vi "FPGACentreReadout.vi"() -> ()   [LabVIEW 2018]
uses:
  State.ctl
  Data.ctl
  <vilib>/rvi/Emulation/niFpgaGetClockAttributes.vi
  <vilib>/rvi/Emulation/niFpgaSctlEmulationGetInTimedLoop.vi
  <vilib>/rvi/Emulation/niFpgaEmulationReportErrorSimple.vi
  <vilib>/rvi/Emulation/niFpgaProcessEmulError.vi
  <vilib>/rvi/eio/common/nirviEmuTemplateMethod_errors.vi
  <vilib>/rvi/Emulation/niFpgaCriticalErrorInLSC.vi
  <vilib>/eio/EIONode/EIONode.xnode
panel:
  out "Boolean":bool
  in  "PowerDown? 3":bool
  out "Data 3":i32
  in  "Gain/ChannelSelect 3":T1(ring)
  out "ConnectorA/DIO4":bool
  out "State 3":T2
  out "Data array3":i32[](array[numeric])
  in  "PowerDown? 2":bool
  out "Data 2":i32
  in  "Gain/ChannelSelect 2":T1(ring)
  out "ConnectorA/DIO2":bool
  out "State 2":T2
  out "Data array 2":i32[](array[numeric])
  out "RawCurrent":u16
  out "RawVoltage":i16
  out "State":T2
  out "ConnectorA/DIO0":bool
  out "Data array":i32[](array[numeric])
  in  "PowerDown?":bool
  out "Data":i32
  in  "Gain/ChannelSelect":T1(ring)
  in  "stop":bool
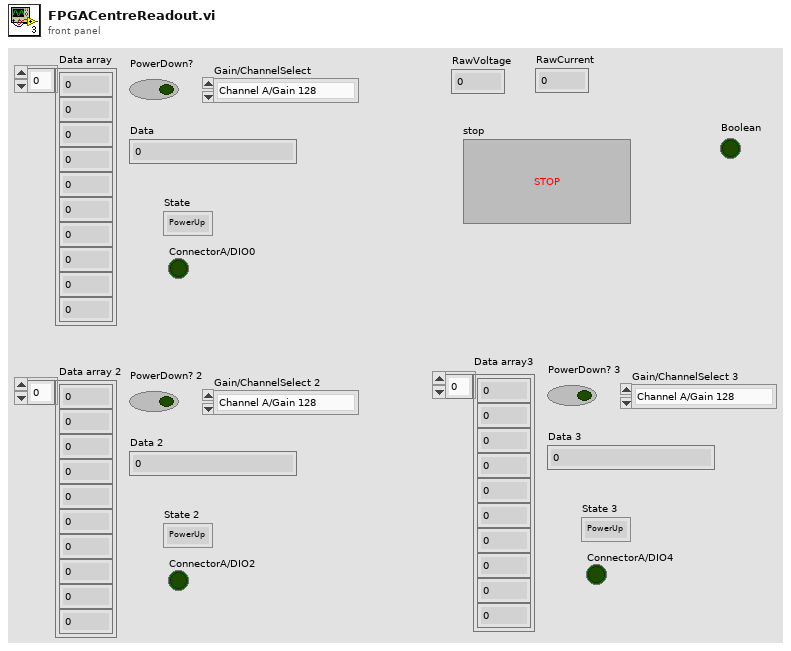
[diagram p1: front panel]
types:
  T1 = enum16{"Channel A/Gain 128", "Channel A/Gain 64", "Channel B/Gain 32"}
  T2 = typedef "State.ctl" = enum16{"PowerUp", "PowerDown", "Gain/ChannelSelect", "ReadData", "ClockLow", "ClockHigh", "ConvertData", "RetrievalReady?"}
  T3 = typedef "Data.ctl" = cluster{"DT":bool, "SCK":bool, "2's Data":i32, "PulseCount":u8, "DelayTime":u8, "Data":i32, "PowerDown?":bool, "Gain/ChannelSelect":enum16{"Channel A/Gain 128", "Channel A/Gain 64", "Channel B/Gain 32"}}
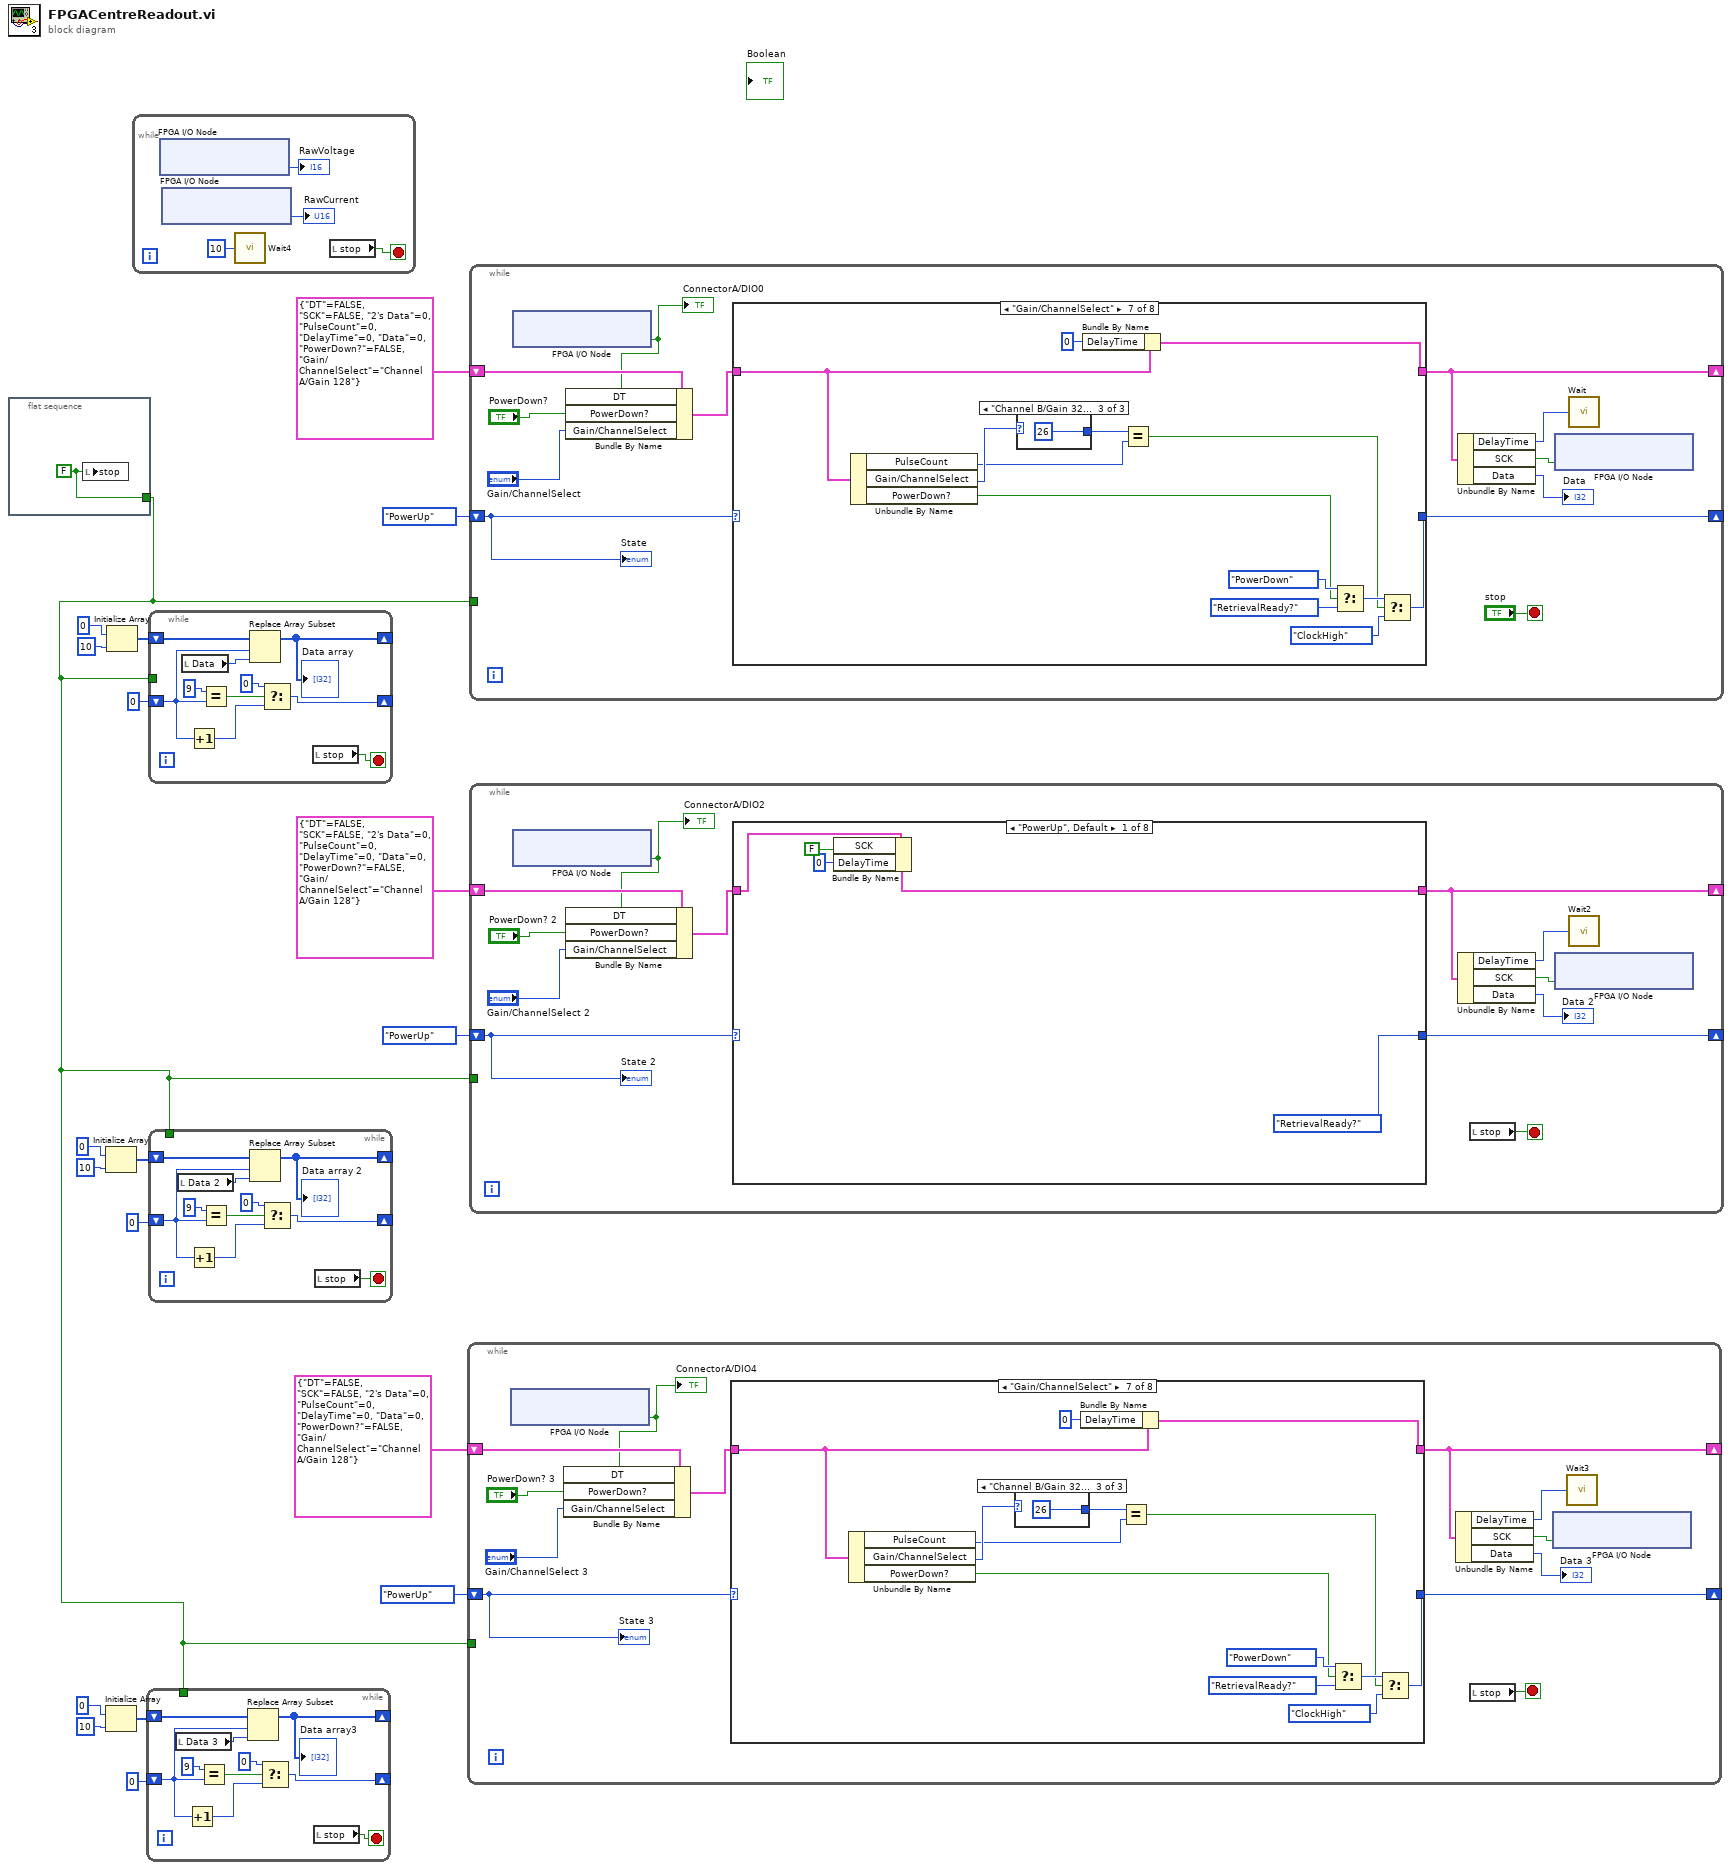
[diagram p0: block diagram]
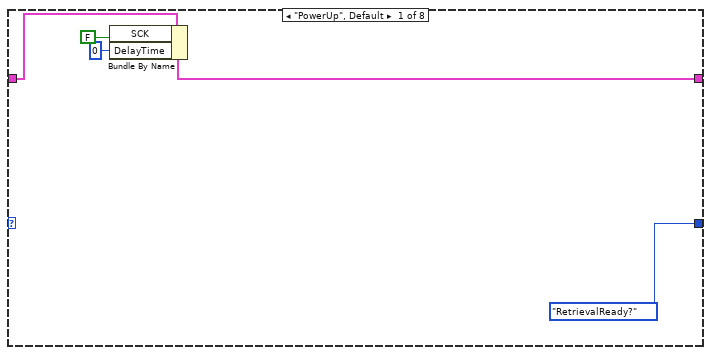
[diagram p2: hidden frame]
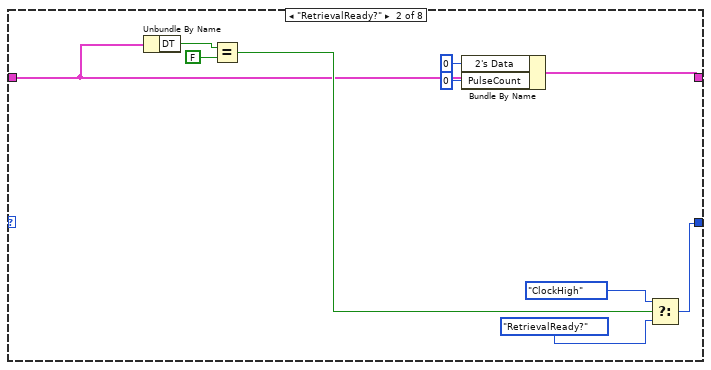
[diagram p3: hidden frame]
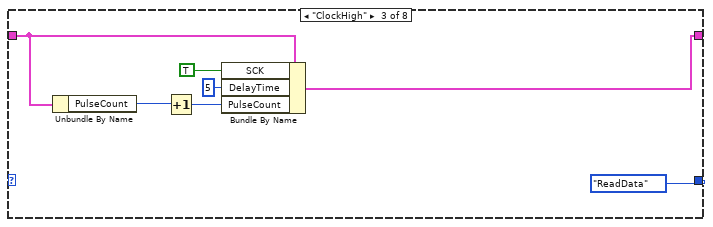
[diagram p4: hidden frame]
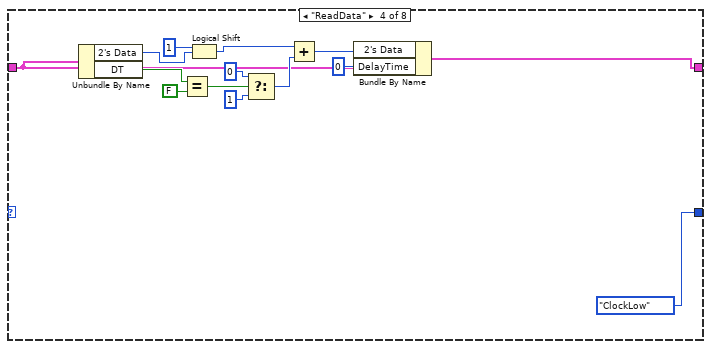
[diagram p5: hidden frame]
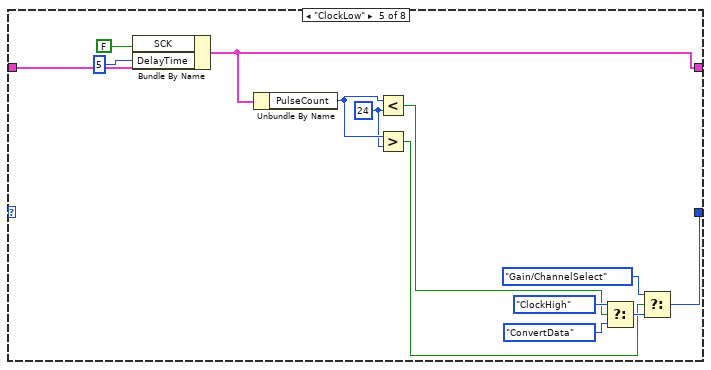
[diagram p6: hidden frame]
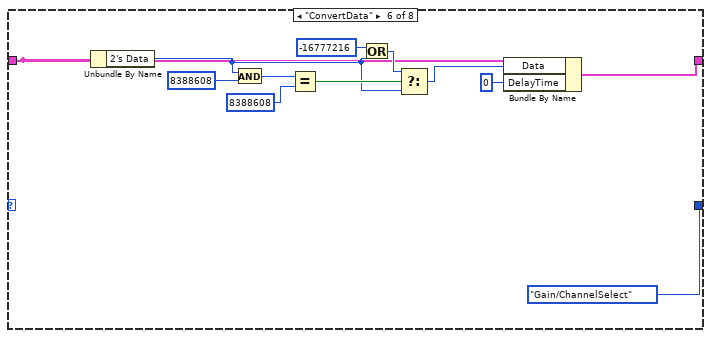
[diagram p7: hidden frame]
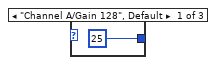
[diagram p8: hidden frame]
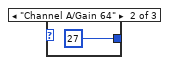
[diagram p9: hidden frame]
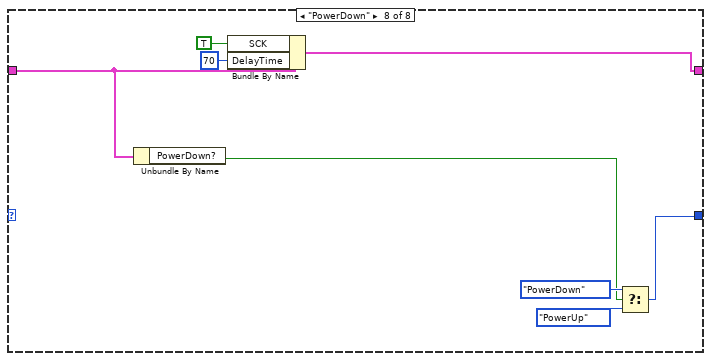
[diagram p10: hidden frame]
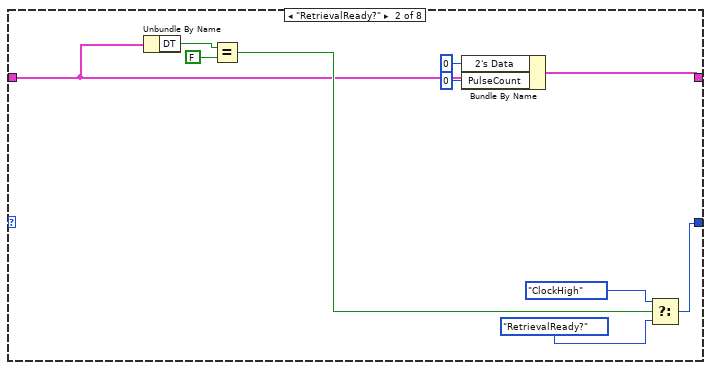
[diagram p11: hidden frame]
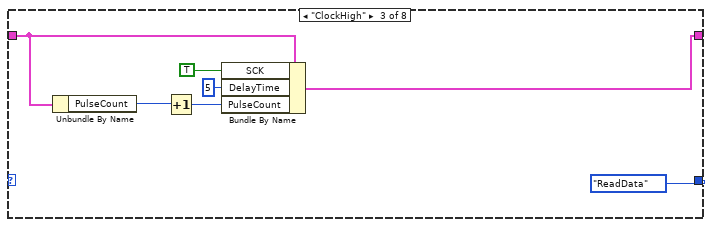
[diagram p12: hidden frame]
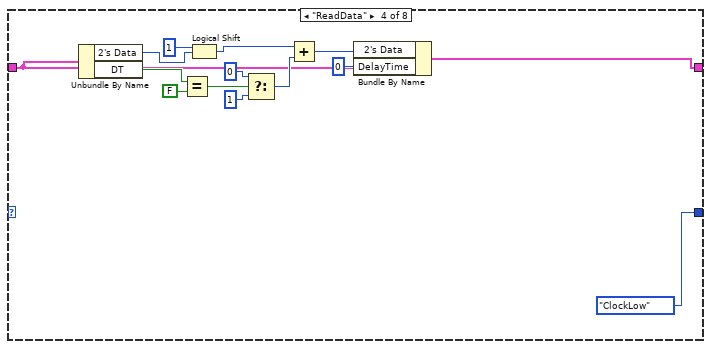
[diagram p13: hidden frame]
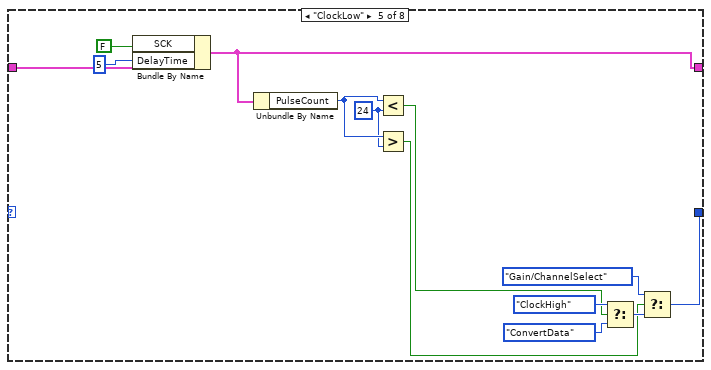
[diagram p14: hidden frame]
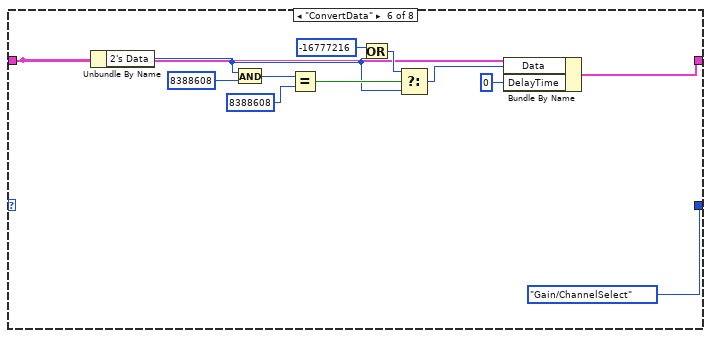
[diagram p15: hidden frame]
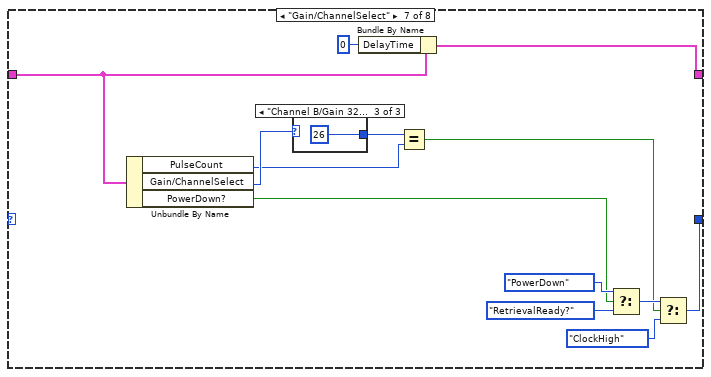
[diagram p16: hidden frame]
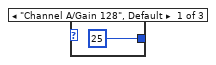
[diagram p17: hidden frame]
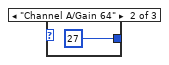
[diagram p18: hidden frame]
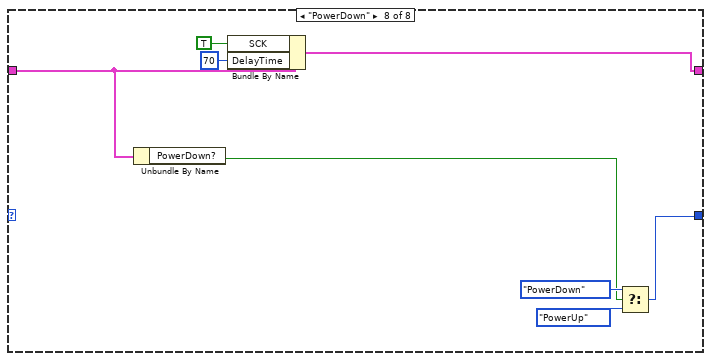
[diagram p19: hidden frame]
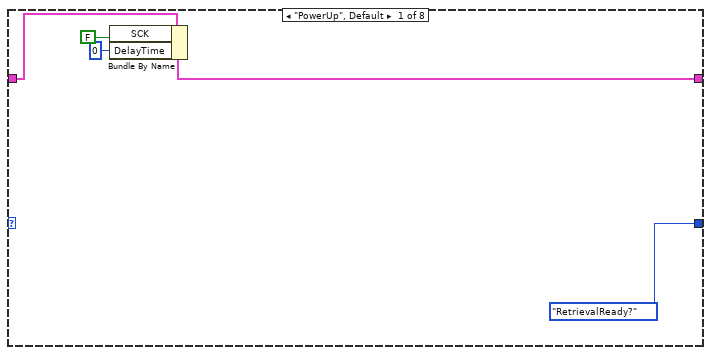
[diagram p20: hidden frame]
diagram:
  n1 = flat-sequence {
    tunnel: [w20] -> w9
    frame #0 {
      w20 = FALSE
      n2 = local write "stop"(w20) -> ()
    }
  }
  n3 = Initialize Array(0 ("Data"), 10 ("dimension size")) -> (w5:i32[])
  n4 = Initialize Array(0 ("Data"), 10 ("dimension size")) -> (w2:i32[])
  n5 = Initialize Array(0 ("Data"), 10 ("dimension size")) -> (w16:i32[])
  n6 = while {
    stop <- w22 stop-if-true
    n7 = xnode "FPGA I/O Node"() -> ("ConnectorC/AI0"=→"RawVoltage":i16)  [unwired: 1 in, 1 out]
    n8 = xnode "FPGA I/O Node"() -> ("ConnectorA/AI0"=→"RawCurrent":u16)  [unwired: 1 in, 1 out]
    n9 = call "Wait4"("Count(mSec)"=u32 10) -> ()  [unwired: 1 out]
    n10 = local read "stop"() -> (w22:bool)
  }
  n11 = while {
    shift-right: [w26] -> _
    shift-left: w2 -> [w27]
    shift-right: [w32] -> _
    shift-left: 0 ("index") -> [w28]
    tunnel: w9 -> [_]
    stop <- w25 stop-if-true
    n12 = local read "Data 3"() -> (w34:i32)
    n13 = Increment(x=w28) -> (x+1=w31:i32)
    n14 = Equal?(x=9, y=w28) -> (x = y?=w29:bool)
    n15 = Replace Array Subset(array=w27, new element=w34, index=w28) -> (w26:i32[])
    "Data array3" <- w26
    n16 = Select(t=0 ("index"), s=w29, f=w31) -> (s? t:f=w32:i32)
    n17 = local read "stop"() -> (w25:bool)
  }
  n18 = while {
    shift-right: [w36] -> _
    shift-left: w16 -> [w37]
    shift-right: [w42] -> _
    shift-left: 0 ("index") -> [w38]
    tunnel: w9 -> [_]
    stop <- w35 stop-if-true
    n19 = local read "Data"() -> (w44:i32)
    n20 = Increment(x=w38) -> (x+1=w41:i32)
    n21 = Equal?(x=9, y=w38) -> (x = y?=w39:bool)
    n22 = Replace Array Subset(array=w37, new element=w44, index=w38) -> (w36:i32[])
    "Data array" <- w36
    n23 = Select(t=0 ("index"), s=w39, f=w41) -> (s? t:f=w42:i32)
    n24 = local read "stop"() -> (w35:bool)
  }
  n25 = while {
    shift-right: [w46] -> _
    shift-left: w5 -> [w47]
    shift-right: [w52] -> _
    shift-left: 0 ("index") -> [w48]
    tunnel: w9 -> [_]
    stop <- w45 stop-if-true
    n26 = local read "Data 2"() -> (w54:i32)
    n27 = Increment(x=w48) -> (x+1=w51:i32)
    n28 = Equal?(x=9, y=w48) -> (x = y?=w49:bool)
    n29 = Replace Array Subset(array=w47, new element=w54, index=w48) -> (w46:i32[])
    "Data array 2" <- w46
    n30 = Select(t=0 ("index"), s=w49, f=w51) -> (s? t:f=w52:i32)
    n31 = local read "stop"() -> (w45:bool)
  }
  n32 = while {
    shift-right: [w58] -> _
    shift-left: T3 {"DT"=FALSE, "SCK"=FALSE, "2's Data"=0, "PulseCount"=0, "DelayTime"=0, "Data"=0, "PowerDown?"=FALSE, "Gain/ChannelSelect"=enum."Channel A/Gain 128"} ("Data") -> [w63]
    shift-right: [w64] -> _
    shift-left: State."PowerUp" ("State") -> [w66]
    tunnel: w9 -> [_]
    stop <- w55 stop-if-true
    n33 = xnode "FPGA I/O Node"() -> ("ConnectorA/DIO4"=w61:bool)  [unwired: 1 in, 1 out]
    "ConnectorA/DIO4" <- w61
    n34 = Bundle By Name(cluster=w63, "DT"=w61, "PowerDown?"="PowerDown? 3", "Gain/ChannelSelect"="Gain/ChannelSelect 3") -> (w62:T3)
    n35 = case shown="\"Gain/ChannelSelect\"" w66 {
      tunnel: w62 -> [w71 w75 w84 w89 w115 w120 w130 w145]
      tunnel: [w69 w74 w88 w91 w110 w119 w129 w151] -> w58
      tunnel: [State."RetrievalReady?" ("State") w77 State."ReadData" ("State") State."ClockLow" ("State") w111 State."Gain/ChannelSelect" ("State") w137 w146] -> w64
      frame "PowerUp", Default {
        n36 = Bundle By Name(cluster=w71, "SCK"=FALSE, "DelayTime"=u8 0) -> (w69:T3)
      }
      frame "RetrievalReady?" {
        n37 = Unbundle By Name(w75) -> ("DT"=w81:bool)
        n38 = Equal?(x=w81, y=FALSE) -> (x = y?=w76:bool)
        n39 = Bundle By Name(cluster=w75, "2's Data"=0, "PulseCount"=u8 0) -> (w74:T3)
        n40 = Select(t=State."ClockHigh" ("State"), s=w76, f=State."RetrievalReady?" ("State")) -> (s? t:f=w77:T2)
      }
      frame "ClockHigh" {
        n41 = Unbundle By Name(w84) -> ("PulseCount"=w83:u8)
        n42 = Increment(x=w83) -> (x+1=w82:u8)
        n43 = Bundle By Name(cluster=w84, "SCK"=TRUE, "DelayTime"=u8 5, "PulseCount"=w82) -> (w88:T3)
      }
      frame "ReadData" {
        n44 = Unbundle By Name(w89) -> ("2's Data"=w102:i32, "DT"=w100:bool)
        n45 = Equal?(x=w100, y=FALSE ("SCK")) -> (x = y?=w98:bool)
        n46 = Logical Shift(y=i16 1, x=w102) -> (x << y=w97:i32)
        n47 = Select(t=0 ("DelayTime"), s=w98, f=1 ("DelayTime")) -> (s? t:f=w94:i32)
        n48 = Add(x=w97, y=w94) -> (x+y=w93:i32)
        n49 = Bundle By Name(cluster=w89, "2's Data"=w93, "DelayTime"=u8 0) -> (w91:T3)
      }
      frame "ClockLow" {
        w104 = u8 24 ("y")
        n50 = Bundle By Name(cluster=w115, "SCK"=FALSE, "DelayTime"=u8 5) -> (w110:T3)
        n51 = Unbundle By Name(w110) -> ("PulseCount"=w105:u8)
        n52 = Less?(x=w105, y=w104) -> (x < y?=w107:bool)
        n53 = Greater?(x=w105, y=w104) -> (0:w103:bool)
        n54 = Select(t=State."ClockHigh" ("State"), s=w107, f=State."ConvertData" ("State")) -> (s? t:f=w106:T2)
        n55 = Select(t=State."Gain/ChannelSelect" ("State"), s=w103, f=w106) -> (s? t:f=w111:T2)
      }
      frame "ConvertData" {
        n56 = Unbundle By Name(w120) -> ("2's Data"=w121:i32)
        n57 = And(x=w121, y=8388608) -> (x .and. y?=w126:i32)
        n58 = Equal?(x=w126, y=8388608) -> (x = y?=w124:bool)
        n59 = Or(x=-16777216 ("y"), y=w121) -> (x .or. y?=w122:i32)
        n60 = Select(t=w122, s=w124, f=w121) -> (s? t:f=w117:i32)
        n61 = Bundle By Name(cluster=w120, "Data"=w117, "DelayTime"=u8 0) -> (w119:T3)
      }
      frame "Gain/ChannelSelect" {
        n62 = Unbundle By Name(w130) -> ("PulseCount"=w133:u8, "Gain/ChannelSelect"=w135:T1, "PowerDown?"=w136:bool)
        n63 = case shown="\"Channel B/Gain 32\"" w135 {
          tunnel: [u8 25 ("PulseCount") u8 27 ("PulseCount") u8 26 ("PulseCount")] -> w134
          frame "Channel A/Gain 128", Default {
          }
          frame "Channel A/Gain 64" {
          }
          frame "Channel B/Gain 32" {
          }
        }
        n64 = Bundle By Name(cluster=w130, "DelayTime"=u8 0) -> (w129:T3)
        n65 = Equal?(x=w134, y=w133) -> (x = y?=w131:bool)
        n66 = Select(t=State."PowerDown" ("State"), s=w136, f=State."RetrievalReady?" ("State")) -> (s? t:f=w132:T2)
        n67 = Select(t=w132, s=w131, f=State."ClockHigh" ("State")) -> (s? t:f=w137:T2)
      }
      frame "PowerDown" {
        n68 = Unbundle By Name(w145) -> ("PowerDown?"=w144:bool)
        n69 = Bundle By Name(cluster=w145, "SCK"=TRUE, "DelayTime"=u8 70) -> (w151:T3)
        n70 = Select(t=State."PowerDown" ("State"), s=w144, f=State."PowerUp" ("State")) -> (s? t:f=w146:T2)
      }
    }
    n71 = Unbundle By Name(w58) -> ("DelayTime"=w65:u8, "SCK"=w57:bool, "Data"=→"Data 3":i32)
    n72 = local read "stop"() -> (w55:bool)
    n73 = xnode "FPGA I/O Node"("ConnectorA/DIO5"=w57) -> ()  [unwired: 1 in, 1 out]
    n74 = call "Wait3"("Count(uSec)"=w65) -> ()  [unwired: 1 out]
    "State 3" <- w66
  }
  n75 = while {
    shift-right: [w154] -> _
    shift-left: T3 {"DT"=FALSE, "SCK"=FALSE, "2's Data"=0, "PulseCount"=0, "DelayTime"=0, "Data"=0, "PowerDown?"=FALSE, "Gain/ChannelSelect"=enum."Channel A/Gain 128"} ("Data") -> [w160]
    shift-right: [w161] -> _
    shift-left: State."PowerUp" ("State") -> [w163]
    tunnel: w9 -> [_]
    stop <- "stop" stop-if-true
    n76 = xnode "FPGA I/O Node"() -> ("ConnectorA/DIO0"=w158:bool)  [unwired: 1 in, 1 out]
    "ConnectorA/DIO0" <- w158
    n77 = Bundle By Name(cluster=w160, "DT"=w158, "PowerDown?"="PowerDown?", "Gain/ChannelSelect"="Gain/ChannelSelect") -> (w159:T3)
    n78 = case shown="\"Gain/ChannelSelect\"" w163 {
      tunnel: w159 -> [w168 w172 w181 w186 w212 w217 w227 w242]
      tunnel: [w166 w171 w185 w188 w207 w216 w226 w248] -> w154
      tunnel: [State."RetrievalReady?" ("State") w174 State."ReadData" ("State") State."ClockLow" ("State") w208 State."Gain/ChannelSelect" ("State") w234 w243] -> w161
      frame "PowerUp", Default {
        n79 = Bundle By Name(cluster=w168, "SCK"=FALSE, "DelayTime"=u8 0) -> (w166:T3)
      }
      frame "RetrievalReady?" {
        n80 = Unbundle By Name(w172) -> ("DT"=w178:bool)
        n81 = Equal?(x=w178, y=FALSE) -> (x = y?=w173:bool)
        n82 = Bundle By Name(cluster=w172, "2's Data"=0, "PulseCount"=u8 0) -> (w171:T3)
        n83 = Select(t=State."ClockHigh" ("State"), s=w173, f=State."RetrievalReady?" ("State")) -> (s? t:f=w174:T2)
      }
      frame "ClockHigh" {
        n84 = Unbundle By Name(w181) -> ("PulseCount"=w180:u8)
        n85 = Increment(x=w180) -> (x+1=w179:u8)
        n86 = Bundle By Name(cluster=w181, "SCK"=TRUE, "DelayTime"=u8 5, "PulseCount"=w179) -> (w185:T3)
      }
      frame "ReadData" {
        n87 = Unbundle By Name(w186) -> ("2's Data"=w199:i32, "DT"=w197:bool)
        n88 = Equal?(x=w197, y=FALSE ("SCK")) -> (x = y?=w195:bool)
        n89 = Logical Shift(y=i16 1, x=w199) -> (x << y=w194:i32)
        n90 = Select(t=0 ("DelayTime"), s=w195, f=1 ("DelayTime")) -> (s? t:f=w191:i32)
        n91 = Add(x=w194, y=w191) -> (x+y=w190:i32)
        n92 = Bundle By Name(cluster=w186, "2's Data"=w190, "DelayTime"=u8 0) -> (w188:T3)
      }
      frame "ClockLow" {
        w201 = u8 24 ("y")
        n93 = Bundle By Name(cluster=w212, "SCK"=FALSE, "DelayTime"=u8 5) -> (w207:T3)
        n94 = Unbundle By Name(w207) -> ("PulseCount"=w202:u8)
        n95 = Less?(x=w202, y=w201) -> (x < y?=w204:bool)
        n96 = Greater?(x=w202, y=w201) -> (0:w200:bool)
        n97 = Select(t=State."ClockHigh" ("State"), s=w204, f=State."ConvertData" ("State")) -> (s? t:f=w203:T2)
        n98 = Select(t=State."Gain/ChannelSelect" ("State"), s=w200, f=w203) -> (s? t:f=w208:T2)
      }
      frame "ConvertData" {
        n99 = Unbundle By Name(w217) -> ("2's Data"=w218:i32)
        n100 = And(x=w218, y=8388608) -> (x .and. y?=w223:i32)
        n101 = Equal?(x=w223, y=8388608) -> (x = y?=w221:bool)
        n102 = Or(x=-16777216 ("y"), y=w218) -> (x .or. y?=w219:i32)
        n103 = Select(t=w219, s=w221, f=w218) -> (s? t:f=w214:i32)
        n104 = Bundle By Name(cluster=w217, "Data"=w214, "DelayTime"=u8 0) -> (w216:T3)
      }
      frame "Gain/ChannelSelect" {
        n105 = Unbundle By Name(w227) -> ("PulseCount"=w230:u8, "Gain/ChannelSelect"=w232:T1, "PowerDown?"=w233:bool)
        n106 = case shown="\"Channel B/Gain 32\"" w232 {
          tunnel: [u8 25 ("PulseCount") u8 27 ("PulseCount") u8 26 ("PulseCount")] -> w231
          frame "Channel A/Gain 128", Default {
          }
          frame "Channel A/Gain 64" {
          }
          frame "Channel B/Gain 32" {
          }
        }
        n107 = Bundle By Name(cluster=w227, "DelayTime"=u8 0) -> (w226:T3)
        n108 = Equal?(x=w231, y=w230) -> (x = y?=w228:bool)
        n109 = Select(t=State."PowerDown" ("State"), s=w233, f=State."RetrievalReady?" ("State")) -> (s? t:f=w229:T2)
        n110 = Select(t=w229, s=w228, f=State."ClockHigh" ("State")) -> (s? t:f=w234:T2)
      }
      frame "PowerDown" {
        n111 = Unbundle By Name(w242) -> ("PowerDown?"=w241:bool)
        n112 = Bundle By Name(cluster=w242, "SCK"=TRUE, "DelayTime"=u8 70) -> (w248:T3)
        n113 = Select(t=State."PowerDown" ("State"), s=w241, f=State."PowerUp" ("State")) -> (s? t:f=w243:T2)
      }
    }
    n114 = Unbundle By Name(w154) -> ("DelayTime"=w162:u8, "SCK"=w153:bool, "Data"=→"Data":i32)
    n115 = xnode "FPGA I/O Node"("ConnectorA/DIO1"=w153) -> ()  [unwired: 1 in, 1 out]
    n116 = call "Wait"("Count(uSec)"=w162) -> ()  [unwired: 1 out]
    "State" <- w163
  }
  n117 = while {
    shift-right: [w252] -> _
    shift-left: T3 {"DT"=FALSE, "SCK"=FALSE, "2's Data"=0, "PulseCount"=0, "DelayTime"=0, "Data"=0, "PowerDown?"=FALSE, "Gain/ChannelSelect"=enum."Channel A/Gain 128"} ("Data") -> [w257]
    shift-right: [w258] -> _
    shift-left: State."PowerUp" ("State") -> [w260]
    tunnel: w9 -> [_]
    stop <- w249 stop-if-true
    n118 = xnode "FPGA I/O Node"() -> ("ConnectorA/DIO2"=w255:bool)  [unwired: 1 in, 1 out]
    "ConnectorA/DIO2" <- w255
    n119 = Bundle By Name(cluster=w257, "DT"=w255, "PowerDown?"="PowerDown? 2", "Gain/ChannelSelect"="Gain/ChannelSelect 2") -> (w256:T3)
    n120 = case shown="\"PowerUp\", Default" w260 {
      tunnel: w256 -> [w265 w269 w278 w283 w309 w314 w324 w339]
      tunnel: [w263 w268 w282 w285 w304 w313 w323 w345] -> w252
      tunnel: [State."RetrievalReady?" ("State") w271 State."ReadData" ("State") State."ClockLow" ("State") w305 State."Gain/ChannelSelect" ("State") w331 w340] -> w258
      frame "PowerUp", Default {
        n121 = Bundle By Name(cluster=w265, "SCK"=FALSE, "DelayTime"=u8 0) -> (w263:T3)
      }
      frame "RetrievalReady?" {
        n122 = Unbundle By Name(w269) -> ("DT"=w275:bool)
        n123 = Equal?(x=w275, y=FALSE) -> (x = y?=w270:bool)
        n124 = Bundle By Name(cluster=w269, "2's Data"=0, "PulseCount"=u8 0) -> (w268:T3)
        n125 = Select(t=State."ClockHigh" ("State"), s=w270, f=State."RetrievalReady?" ("State")) -> (s? t:f=w271:T2)
      }
      frame "ClockHigh" {
        n126 = Unbundle By Name(w278) -> ("PulseCount"=w277:u8)
        n127 = Increment(x=w277) -> (x+1=w276:u8)
        n128 = Bundle By Name(cluster=w278, "SCK"=TRUE, "DelayTime"=u8 5, "PulseCount"=w276) -> (w282:T3)
      }
      frame "ReadData" {
        n129 = Unbundle By Name(w283) -> ("2's Data"=w296:i32, "DT"=w294:bool)
        n130 = Equal?(x=w294, y=FALSE ("SCK")) -> (x = y?=w292:bool)
        n131 = Logical Shift(y=i16 1, x=w296) -> (x << y=w291:i32)
        n132 = Select(t=0 ("DelayTime"), s=w292, f=1 ("DelayTime")) -> (s? t:f=w288:i32)
        n133 = Add(x=w291, y=w288) -> (x+y=w287:i32)
        n134 = Bundle By Name(cluster=w283, "2's Data"=w287, "DelayTime"=u8 0) -> (w285:T3)
      }
      frame "ClockLow" {
        w298 = u8 24 ("y")
        n135 = Bundle By Name(cluster=w309, "SCK"=FALSE, "DelayTime"=u8 5) -> (w304:T3)
        n136 = Unbundle By Name(w304) -> ("PulseCount"=w299:u8)
        n137 = Less?(x=w299, y=w298) -> (x < y?=w301:bool)
        n138 = Greater?(x=w299, y=w298) -> (0:w297:bool)
        n139 = Select(t=State."ClockHigh" ("State"), s=w301, f=State."ConvertData" ("State")) -> (s? t:f=w300:T2)
        n140 = Select(t=State."Gain/ChannelSelect" ("State"), s=w297, f=w300) -> (s? t:f=w305:T2)
      }
      frame "ConvertData" {
        n141 = Unbundle By Name(w314) -> ("2's Data"=w315:i32)
        n142 = And(x=w315, y=8388608) -> (x .and. y?=w320:i32)
        n143 = Equal?(x=w320, y=8388608) -> (x = y?=w318:bool)
        n144 = Or(x=-16777216 ("y"), y=w315) -> (x .or. y?=w316:i32)
        n145 = Select(t=w316, s=w318, f=w315) -> (s? t:f=w311:i32)
        n146 = Bundle By Name(cluster=w314, "Data"=w311, "DelayTime"=u8 0) -> (w313:T3)
      }
      frame "Gain/ChannelSelect" {
        n147 = Unbundle By Name(w324) -> ("PulseCount"=w327:u8, "Gain/ChannelSelect"=w329:T1, "PowerDown?"=w330:bool)
        n148 = case shown="\"Channel B/Gain 32\"" w329 {
          tunnel: [u8 25 ("PulseCount") u8 27 ("PulseCount") u8 26 ("PulseCount")] -> w328
          frame "Channel A/Gain 128", Default {
          }
          frame "Channel A/Gain 64" {
          }
          frame "Channel B/Gain 32" {
          }
        }
        n149 = Bundle By Name(cluster=w324, "DelayTime"=u8 0) -> (w323:T3)
        n150 = Equal?(x=w328, y=w327) -> (x = y?=w325:bool)
        n151 = Select(t=State."PowerDown" ("State"), s=w330, f=State."RetrievalReady?" ("State")) -> (s? t:f=w326:T2)
        n152 = Select(t=w326, s=w325, f=State."ClockHigh" ("State")) -> (s? t:f=w331:T2)
      }
      frame "PowerDown" {
        n153 = Unbundle By Name(w339) -> ("PowerDown?"=w338:bool)
        n154 = Bundle By Name(cluster=w339, "SCK"=TRUE, "DelayTime"=u8 70) -> (w345:T3)
        n155 = Select(t=State."PowerDown" ("State"), s=w338, f=State."PowerUp" ("State")) -> (s? t:f=w340:T2)
      }
    }
    n156 = Unbundle By Name(w252) -> ("DelayTime"=w259:u8, "SCK"=w251:bool, "Data"=→"Data 2":i32)
    n157 = local read "stop"() -> (w249:bool)
    n158 = xnode "FPGA I/O Node"("ConnectorA/DIO3"=w251) -> ()  [unwired: 1 in, 1 out]
    n159 = call "Wait2"("Count(uSec)"=w259) -> ()  [unwired: 1 out]
    "State 2" <- w260
  }
